vi "Analog Receive String.vi"(0 "System no.":i32=1 min=1 step=1, 1 "String in":string, 2 "Read/Write (T)":bool, 3 "Ini":bool, 5 "error in":errorcluster) -> (14 "String out":string, 19 "error out":errorcluster)   [LabVIEW 2020]
doc: "This VI works as an old style global variable for String out.\n\nValid for Analog Systems (but must be present for all other systems, too)"
panel:
  out "Strings out":string[](array[string])
  # "This VI works as an old style global variable for String out."
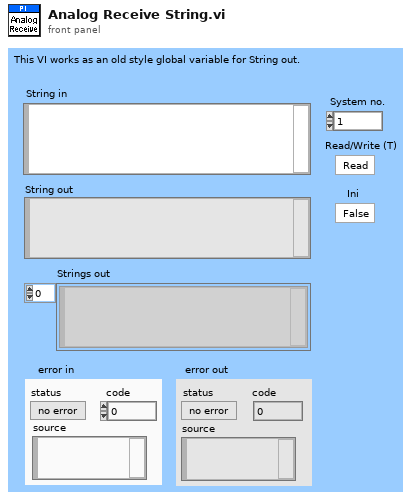
[diagram p1: front panel]
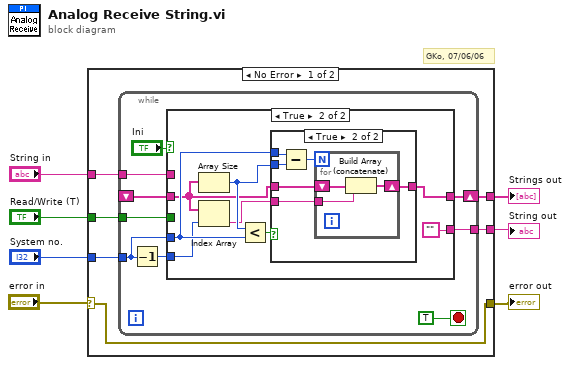
[diagram p0: block diagram]
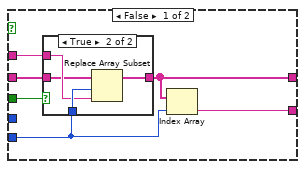
[diagram p2: hidden frame]
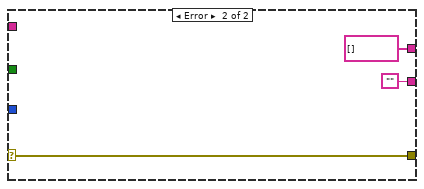
[diagram p5: hidden frame]
diagram:
  # "GKo, 07/06/06"
  n1 = case shown="No Error" "error in" {
    selector: "error in" -> [w8 w54]
    tunnel: "String in" -> [w13 _]
    tunnel: "Read/Write (T)" -> [w12 _]
    tunnel: "System no." -> [w11 _]
    tunnel: [w10 string[] []] -> w3
    tunnel: [w9 "" ("String in")] -> w2
    tunnel: [w8 w54] -> w1
    frame No Error {
      n2 = while {
        shift-right: [w18] -> w10
        shift-left: _ -> [w19]
        tunnel: w12 -> [w21]
        tunnel: w13 -> [w20]
        tunnel: w11 -> [w14]
        tunnel: [w16] -> w9
        stop <- TRUE stop-if-true
        n3 = Decrement(x=w14) -> (x-1=w17:i32)
        n4 = case shown="True" "Ini" {
          tunnel: w21 -> [w28 _]
          tunnel: w20 -> [w27 _]
          tunnel: w19 -> [w26 w39]
          tunnel: [w25 w36] -> w18
          tunnel: w17 -> [w24 w38]
          tunnel: [w23 "" ("String in")] -> w16
          tunnel: w14 -> [_ w41]
          frame False {
            n5 = case shown="True" w28 {
              tunnel: w27 -> [_ w32]
              tunnel: w24 -> [_ w33]
              tunnel: w26 -> [w29 w31]
              tunnel: [w29 w30] -> w25
              frame False {
              }
              frame True {
                n6 = Replace Array Subset(array=w31, new element=w32, index=w33) -> (w30:string[])
              }
            }
            n7 = Index Array(array=w25, index=w24) -> (element=w23:string)
          }
          frame True {
            n8 = Array Size(array=w39) -> (size(s)=w40:i32)
            n9 = Index Array(array=w39, index=w38) -> (element=w37:string)
            n10 = Less?(x=w40, y=w41) -> (x < y?=w34:bool)
            n11 = case shown="True" w34 {
              tunnel: w41 -> [_ w47]
              tunnel: w40 -> [_ w46]
              tunnel: w39 -> [w42 w45]
              tunnel: w37 -> [_ w44]
              tunnel: [w42 w43] -> w36
              frame False {
              }
              frame True {
                n12 = Subtract(x=w47, y=w46) -> (x-y=w48:i32)
                n13 = for {
                  N: w48 -> [_]
                  shift-right: [w51] -> w43
                  shift-left: w45 -> [w50]
                  tunnel: w44 -> [w49]
                  n14 = Build Array (concatenate)(w50, w49) -> (w51:string[])
                }
              }
            }
          }
        }
      }
    }
    frame Error {
    }
  }
  "Strings out" <- w3
  "String out" <- w2
  "error out" <- w1
